vi "finishPrepareKickoffEnemyPlayVSS.vi"(8 "error in (no error)":errorcluster, 10 "Game in":refnum<class "Game.lvclass">, 11 "PrepareKickoffEnemyPlayVSS in":refnum<class "PrepareKickoffEnemyPlayVSS.lvclass">) -> (0 "error out":errorcluster, 2 "Boolean":bool, 3 "PrepareKickoffEnemyPlayVSS out":refnum<class "PrepareKickoffEnemyPlayVSS.lvclass">)   [LabVIEW 2020, in "PrepareKickoffEnemyPlayVSS.lvclass"]
uses:
  PrepareKickoffEnemyPlayVSS.lvclass
  Game_class/Game.lvclass
  Game_class/Game.lvclass/Game.ctl
  Game_class/Read Referee.vi
  Referee_class/Referee.lvclass
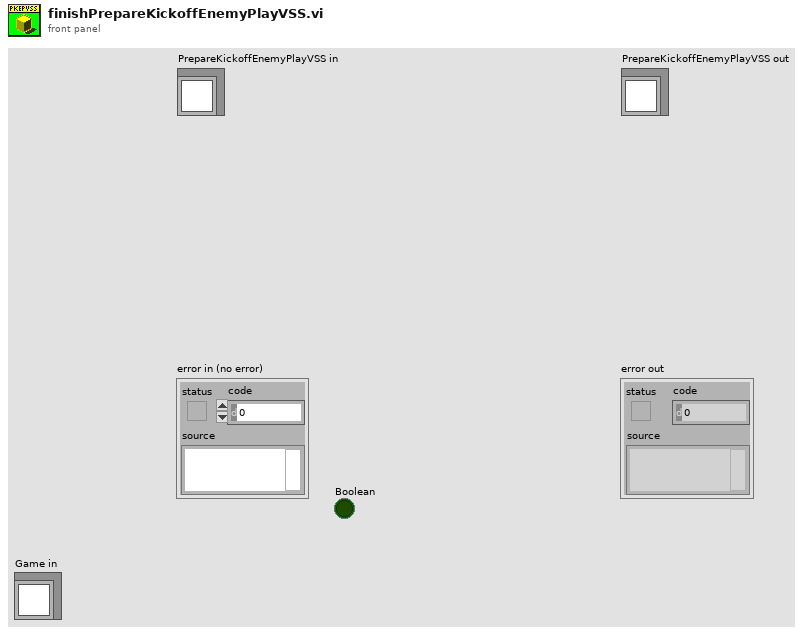
[diagram p1: front panel]
types:
  T1 = enum16{"AUTO", "GAME_ON", "STOP", "KICKOFF", "FREE_BALL", "GOAL_KICK", "PENALTY_KICK", "FREE_KICK"}
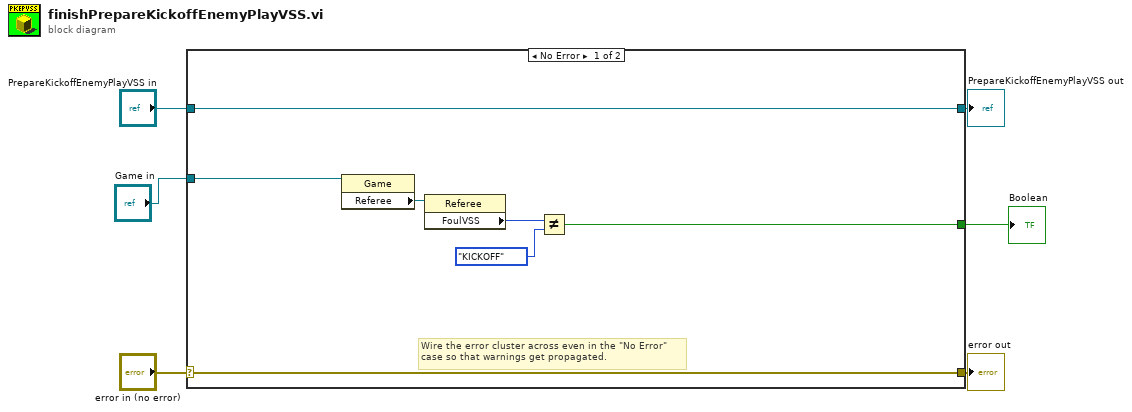
[diagram p0: block diagram]
diagram:
  n1 = case shown="No Error" "error in (no error)" {
    selector: "error in (no error)" -> [w12 w15]
    tunnel: [w12 w15] -> w5
    tunnel: [w13 w14] -> w3
    tunnel: "PrepareKickoffEnemyPlayVSS in" -> [w13 w14]
    tunnel: "Game in" -> [w8 _]
    tunnel: [w7 _] -> w1
    frame No Error {
      # "Wire the error cluster across even in the \"No Error\"\ncase so that warnings get propagated."
      n2 = property class="Game"(reference=w8) -> ("Referee"=w11:refnum<class "Referee.lvclass">)  [unwired: 1 in, 2 out]
      n3 = property class="Referee"(reference=w11) -> ("FoulVSS"=w10:T1)  [unwired: 1 in, 2 out]
      n4 = Not Equal?(x=w10, y=T1."KICKOFF" ("FoulVSS")) -> (x != y?=w7:bool)
    }
    frame Error {
    }
  }
  "error out" <- w5
  "PrepareKickoffEnemyPlayVSS out" <- w3
  "Boolean" <- w1
